vi "Save Analysis Result Histogram Color Grade.vi"(8 "error in (no error)":errorcluster, 9 "Include Histogram Statistics (F: Disable)":bool, 10 "Include Color Grade Data (F: Disable)":bool, 11 "VISA resource name":refnum<visa-resource-name>) -> (0 "error out":errorcluster, 3 "VISA resource name out":refnum<visa-resource-name>)   [LabVIEW 2015, in "Agilent 2000 3000 X-Series.lvlib"]
doc: "Enables or Disables including color grade and histogram data in the saved file. Call <b>Save Analysis Result</b> after this VI to save to a file.\n\n<b>Note:</b>\nThis VI is specific to the 6000-X, DSO/MSO X 3000 G Series oscilloscopes. These features are not available on other models."
uses:
  Agilent 2000 3000 X-Series.lvlib
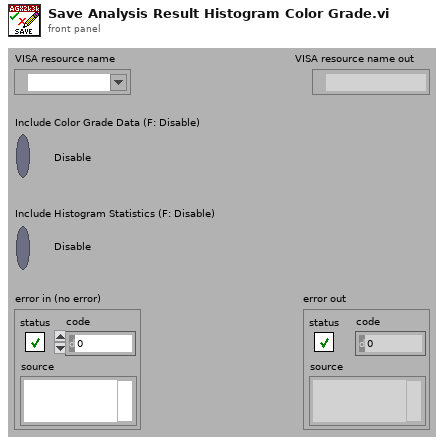
[diagram p1: front panel]
types:
  T1 = typedef "Agilent 2000 3000 X-Series.lvlib/Extended User Data.ctl" = cluster{"X-Series Mode":u16, "Acquisition Type (0: Normal)":i32}
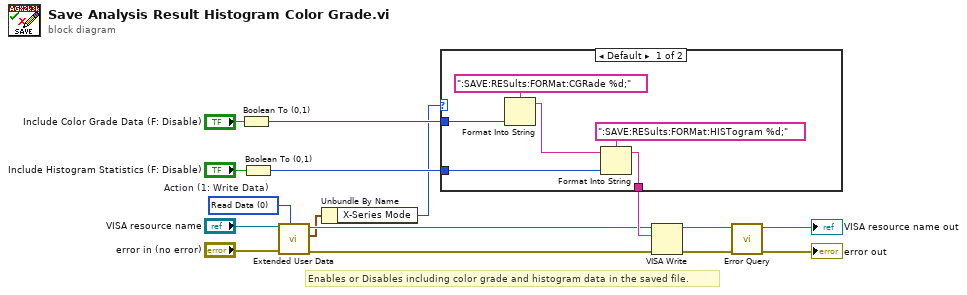
[diagram p0: block diagram]
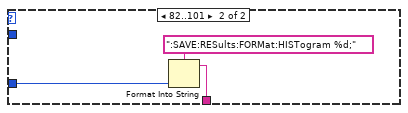
[diagram p2: hidden frame]
diagram:
  w3 = 0 items=["Read Data", "Write Data", "Clear Data", "Clear ALL Data"]  # Action (1: Write Data)
  # "Enables or Disables including color grade and histogram data in the saved file."
  n1 = Boolean To (0,1)(Boolean="Include Color Grade Data (F: Disable)") -> (0, 1=w14:i16)
  n2 = Boolean To (0,1)(Boolean="Include Histogram Statistics (F: Disable)") -> (0, 1=w13:i16)
  n3 = call "Extended User Data.vi"("Action (1: Write Data)"=w3, "error in (no error)"="error in (no error)", "VISA resource name in"="VISA resource name") -> ("error out"=w4:errorcluster, "User Data Out"=w2:T1, "VISA resource name out"=w5:refnum<visa-resource-name>)  [unwired: 6 in]
  n4 = Unbundle By Name(w2) -> ("X-Series Mode"=w1:u16)
  n5 = case shown="Default" w1 {
    tunnel: w14 -> [w22 _]
    tunnel: w13 -> [w20 w25]
    tunnel: [w18 w23] -> w12
    frame Default {
      n6 = Format Into String(format string=":SAVE:RESults:FORMat:CGRade %d;", w22) -> (resulting string=w17:string)  [unwired: 2 in, 1 out]
      n7 = Format Into String(format string=":SAVE:RESults:FORMat:HISTogram %d;", initial string=w17, w20) -> (resulting string=w18:string)  [unwired: 1 in, 1 out]
    }
    frame 82..101 {
      n8 = Format Into String(format string=":SAVE:RESults:FORMat:HISTogram %d;", w25) -> (resulting string=w23:string)  [unwired: 2 in, 1 out]
    }
  }
  n9 = VISA Write(VISA resource name=w5, write buffer=w12, error in (no error)=w4) -> (VISA resource name out=w11:refnum<visa-resource-name>, error out=w10:errorcluster)  [unwired: 1 out]
  n10 = call "Error Query.vi"("error in (no error)"=w10, "VISA resource name"=w11) -> ("error out"=→"error out":errorcluster, "VISA resource name out"=→"VISA resource name out":refnum<visa-resource-name>)  [unwired: 6 in, 2 out]
